vi "Read formattedOutputData.vi"(11 "ILC in":refnum<class "ILC.lvclass">) -> (2 "formattedOutputData":string, 3 "ILC out":refnum<class "ILC.lvclass">)   [LabVIEW 2013]
uses:
  <userlib>/Common/ILC/ILC/ILC.lvclass
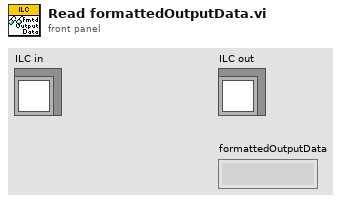
[diagram p1: front panel]
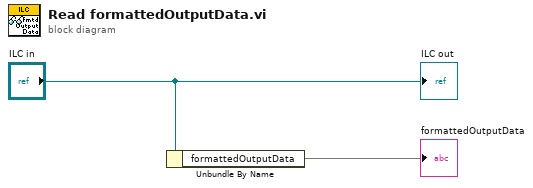
[diagram p0: block diagram]
diagram:
  n1 = Unbundle By Name("ILC in") -> ("formattedOutputData"=→"formattedOutputData")
  "ILC out" <- "ILC in"
